vi "PayloadToJSON.vi"(8 "error in":errorcluster, 11 "Payload":string) -> (0 "error out":errorcluster, 1 "JSON string":string, 2 "UNIX Timestamp":string, 3 "Unix Time (s)":i64)   [LabVIEW 2024]
uses:
  Controls/PayloadCluster.ctl
  <vilib>/LabVIEW Open Source Project/Epoch Date & Time/epoch.UNIX/Epoch.UNIX.lvclass
  <vilib>/LabVIEW Open Source Project/Epoch Date & Time/Get Epoch Time.vi
panel:
  in  "Cluster":T1
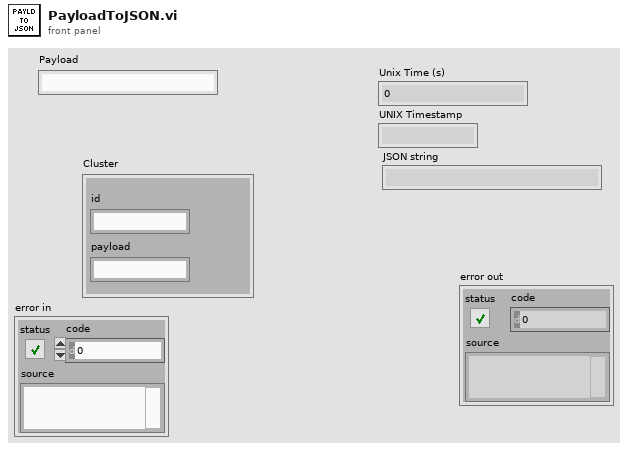
[diagram p1: front panel]
types:
  T1 = typedef "PayloadCluster.ctl" = cluster{"id":string, "payload":string}
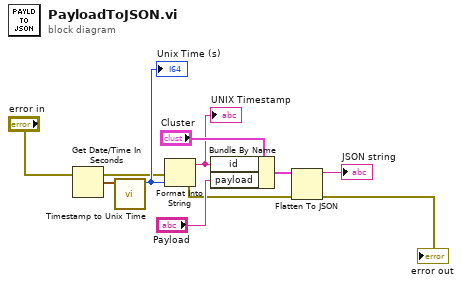
[diagram p0: block diagram]
diagram:
  n1 = Get Date/Time In Seconds() -> (seconds since 1Jan1904=w9:timestamp)
  n2 = call <vilib>:"Timestamp to Unix Time.vi"("Timestamp (now)"=w9) -> ("Unix Time (s)"=w10:i64)  [unwired: 9 in, 1 out]
  "Unix Time (s)" <- w10
  n3 = Format Into String(error in="error in", w10) -> (resulting string=w6:string, error out=w3:errorcluster)  [unwired: 2 in]
  "UNIX Timestamp" <- w6
  n4 = Bundle By Name(cluster="Cluster", "id"=w6, "payload"="Payload") -> (w8:T1)
  n5 = Flatten To JSON(anything=w8, error in (no error)=w3) -> (JSON string=→"JSON string":string, 11:→"error out":errorcluster)  [unwired: 1 in]
